vi "Generate String.vi"(8 "error in (no error)":errorcluster, 11 "object in":refnum<class "Variable_Declaration.lvclass">) -> (0 "error out":errorcluster, 2 "resulting string":string, 3 "object out":refnum<class "Variable_Declaration.lvclass">)   [LabVIEW 2017, in "Variable_Declaration.lvclass"]
uses:
  Variable_Declaration.lvclass
  Variable_Declaration.lvclass/Variable_Declaration.ctl
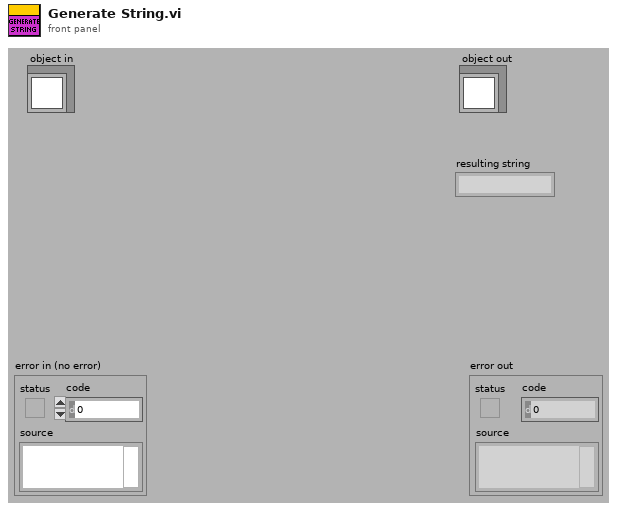
[diagram p1: front panel]
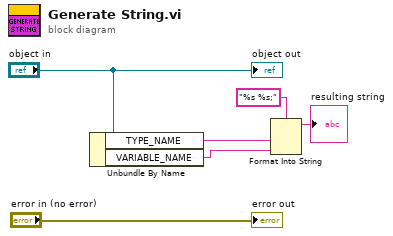
[diagram p0: block diagram]
diagram:
  n1 = Unbundle By Name("object in") -> ("TYPE_NAME"=w3:string, "VARIABLE_NAME"=w2:string)
  n2 = Format Into String(format string="%s %s;", w3, w2) -> (resulting string=→"resulting string":string)  [unwired: 2 in, 1 out]
  "error out" <- "error in (no error)"
  "object out" <- "object in"
